vi "Check_Data.vi"(8 "error constant":errorcluster, 10 "UI Data":T2={"Script_Tree"=refnum, "Scripts"=[], "ScriptDetails"={"Script Name"="", "Steps"=[]}, "Current Step"={"StepName"="", "StepDetails"="", "Type"=enum."RELAY_CHANNEL_WRITE"}, "ScriptName"="", "StepName"="", "Children Symbols"=[], "Parrent Symbol"=[], "Configurations:"="", "Config"="", "Scriptno."=0, "PS_Write"={"Set_parameter"=0, "VOLTAGE"="", "CURRENT"="", "OUTPUT"=FALSE, "Delay"=FALSE, "Delay time"=0.0}, "DMM_CONFIG"={"CONFIG PARAMETER"=0, "AUTO RANGE"=FALSE, "RANGE"="", "Delay"=FALSE, "Delay time"=0.0}, "READ_DATAS"={"EQUIPMENT"=0, "PARAMETER"=0, "LSL"=0.0, "USL"=0.0, "RESULT"="", "UNIT"="", "Delay"=FALSE, "Delay time"=0.0}, "Set_Channel_Relay"={"Relay_CH_Array"=[]}, "DAQ_Config"={"AUTO RANGE"=FALSE, "CHANNEL LIST"="", "SELECT Card"=0, "SELECT SLOT"=0, "Function"=0}, "CAN_MSGs_Write"={"Scaling Factor"=1, "Physical value"=0.0, "CAN_Frames"={"CAN_ID"=0, "MSGTYPE"=128, "Payload"=[], "Length"=0}, "Offset value"=0.0, "Framing datas"=[], "CAN_Frame Enable"=FALSE, "Add Signal"=FALSE, "Delete Signal"=FALSE, "Signal Values"=[], "Time(ms)"=0.0, "Repetition"=FALSE, "Delay"=FALSE, "Delay time"=0.0}, "CAN_Read"={"Database"="", "Signal"="", "BYTES"=[], "ReadPayload"=[], "String_Data"="", "ReadValue"=0.0, "CANID"=0, "SERVICE ID"=0, "SUB-SERVICE ID"=0, "DELAY "=FALSE, "Delay time(ms)"=0.0}, "Camera"={"Trigger"=FALSE, "Prog No."="", "Delay"=FALSE, "Delay time"=0.0, "Storage"="", "Col no."="", "Row no."=""}, "Tab Control"=refnum, "MCU Flashing"={"Result Path"=path "", "Result"=""}, "Noeway_Flashing"={"Neoway_Firmware"=path "", "RESULT STRING"="", "Delay"=FALSE, "Delay time"=0.0}, "SSL"={"SSL_EXE"=path "", "RESULT STRING"="", "Delay"=FALSE, "Delay time"=0.0}} {"CAN_Read"."SUB-SERVICE ID" format="%.0x"; "CAN_Read"."SERVICE ID" format="%.0x"; "CAN_Read"."CANID" format="%.0x"; "CAN_Read"."ReadPayload" format="%.0x"; "CAN_MSGs_Write"."CAN_Frames"."Payload" format="%.0x"; "CAN_MSGs_Write"."CAN_Frames"."MSGTYPE" items=["STATUS"=128, "EXTENDED"=2, "RTR"=1, "DATA MSG"=0]; "CAN_MSGs_Write"."CAN_Frames"."CAN_ID" format="%.0x"; "DAQ_Config"."Function" items=["Voltage DC", "Voltage AC", "Current DC", "Current AC", "Resistance", "4-wire Resistance", "Diode", "Capacitance", "Temperature", "Continuity", "Frequency", "Period", "Voltage Ratio", "Digitize Voltage", "Digitize Current"]; "DAQ_Config"."SELECT SLOT" items=["Slot 1", "Slot 2"]; "DAQ_Config"."SELECT Card" items=["7708", "7700"]; "Set_Channel_Relay"."Relay_CH_Array"."OUTPUT_Relay_Channels" items=["CONN_SUPPLY_%d_FCT", "HB_CONN_%d_FCT", "L_IND_CONN_%d_FCT", "R_IND_CONN_%d_FCT", "SW1_%d_FCT", "SW2_%d_FCT", "CAN_H_%d_FCT", "CAN_L_%d_FCT", "CYLINDER_ON/OFF_%d_FCT", "SPARE_1_%d_FCT", "SPARE_2_%d_FCT", "Tower Red", "Tower Amber", "Tower Green", "Tower Buzzer", "SLIMRELAY_DUT_%d_FCT", "GND_DMM_%d_EOL", "CAN_H_RES_%d_EOL", "CAN_L_RES_%d_EOL", "L_IND_RES_%d_EOL", "R_IND_RES_%d_EOL", "HB_CONN_DMM_%d_EOL", "14V_RES_%d_EOL", "CAN_L_(DMM-)_%d_EOL", "CAN_H_%d_EOL", "CAN_L_%d_EOL", "14V_%d_EOL", "GND_%d_EOL", "HB_CONN_%d_EOL", "L_IND_%d_EOL", "R_IND_%d_EOL", "CYLINDER_DUT_%d_EOL", "CYL_PB_1_%d_EOL", "CYL_PB_2_%d_EOL", "DUT_PASS_%d_EOL", "DUT_FAIL_%d_EOL", "SPARE1_%d_EOL", "Tower Red_EOL", "Tower Amber_EOL", "Tower Green_EOL", "Tower Buzzer_EOL"]; "READ_DATAS"."PARAMETER" items=["SET_VOLTAGE", "SET_CURRENT", "OUTPUT VOLTAGE", "OUTPUT CURRENT", "RESISTANCE", "OUTPUT POWER", "CAMERA", "SSL_Check"]; "READ_DATAS"."EQUIPMENT" items=["POWER SUPPLY", "DMM", "DAQ", "CAMERA"]; "DMM_CONFIG"."CONFIG PARAMETER" items=["VOLTAGE", "CURRENT", "RESISTANCE", "POWER"]; "PS_Write"."Set_parameter" items=["Set_Voltage", "Set_current", "Output"]}) -> (0 "error constant 2":errorcluster, 3 "Fail?":bool)   [LabVIEW 2024, in "Setting_Screen.lvlib"]
uses:
  Setting_Screen.lvlib
  controls/Setting_Screen UI Data.ctl
  ScriptDetails.ctl
  CurrentStep.ctl
  StepType.ctl
  PS_WRITE.ctl
  PS_set.ctl
  DMM_CONFIG.ctl
  READ_DATAS.ctl
  READ_EQP.ctl
  READ_PARA.ctl
  Relay_Channel_Array.ctl
  Common_plc_DOs.ctl
  DAQ_Config.ctl
  PCANusb_DTU/support/CAN_MSGs.ctl
  PCANusb_DTU/support/CAN_Frames_ctrl.ctl
  PCANusb_DTU/support/Framing datas.ctl
  PCANusb_DTU/support/CAN_Read.ctl
  Camera.ctl
  Steptab.ctl
  MCU_Flashing/support/MCU_ctrl.ctl
  Neoway ctl.ctl
  SSL.ctl
  LOAD_WRITE.ctl
  PCANusb_DTU/PCANusb_DTU.lvlib
  MCU_Flashing/MCU_Flashing.lvlib
panel:
  out "Relay_CH_Array":cluster{"OUTPUT_PLC":T1, "On/Off":bool}[](array[cluster]) {"OUTPUT_PLC" items=["CONN_SUPPLY_%d_FCT", "HB_CONN_%d_FCT", "L_IND_CONN_%d_FCT", "R_IND_CONN_%d_FCT", "SW1_%d_FCT", "SW2_%d_FCT", "CAN_H_%d_FCT", "CAN_L_%d_FCT", "CYLINDER_ON/OFF_%d_FCT", "SPARE_1_%d_FCT", "SPARE_2_%d_FCT", "Tower Red", "Tower Amber", "Tower Green", "Tower Buzzer", "SLIMRELAY_DUT_%d_FCT", "GND_DMM_%d_EOL", "CAN_H_RES_%d_EOL", "CAN_L_RES_%d_EOL", "L_IND_RES_%d_EOL", "R_IND_RES_%d_EOL", "HB_CONN_DMM_%d_EOL", "14V_RES_%d_EOL", "CAN_L_(DMM-)_%d_EOL", "CAN_H_%d_EOL", "CAN_L_%d_EOL", "14V_%d_EOL", "GND_%d_EOL", "HB_CONN_%d_EOL", "L_IND_%d_EOL", "R_IND_%d_EOL", "CYLINDER_DUT_%d_EOL", "CYL_PB_1_%d_EOL", "CYL_PB_2_%d_EOL", "DUT_PASS_%d_EOL", "DUT_FAIL_%d_EOL", "SPARE1_%d_EOL", "Tower Red_EOL", "Tower Amber_EOL", "Tower Green_EOL", "Tower Buzzer_EOL"]}
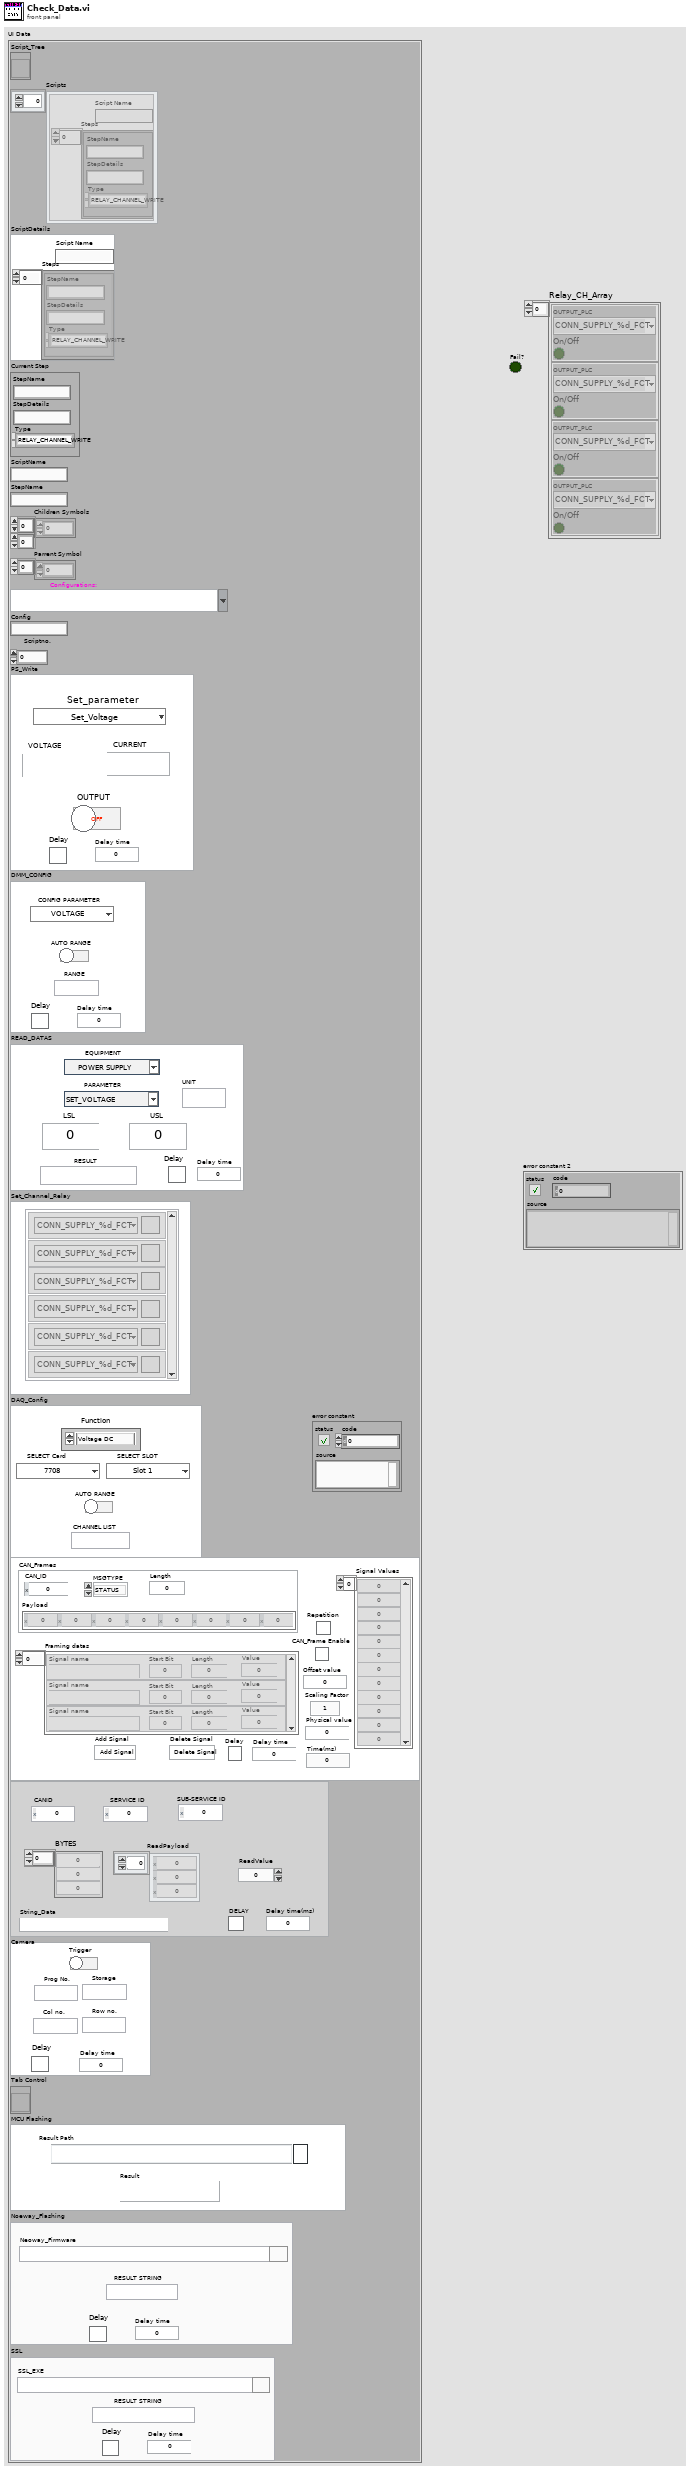
[diagram p1: front panel]
types:
  T1 = typedef "Setting_Screen.lvlib/Common_plc_DOs.ctl" = u16
  T2 = typedef "Setting_Screen.lvlib/Setting_Screen UI Data.ctl" = cluster{"Script_Tree":refnum<vi>, "Scripts":T3[], "ScriptDetails":T3, "Current Step":T4, "ScriptName":string, "StepName":string, "Children Symbols":i32[][], "Parrent Symbol":i32[], "Configurations:":string, "Config":string, "Scriptno.":i32, "PS_Write":T6, "DMM_CONFIG":T8, "READ_DATAS":T9, "Set_Channel_Relay":T12, "DAQ_Config":T13, "CAN_MSGs_Write":T14, "CAN_Read":T17, "Camera":T18, "Tab Control":refnum<vi>, "MCU Flashing":T19, "Noeway_Flashing":T20, "SSL":T21}
  T3 = typedef "Setting_Screen.lvlib/ScriptDetails.ctl" = cluster{"Script Name":string, "Steps":T4[]}
  T4 = typedef "Setting_Screen.lvlib/CurrentStep.ctl" = cluster{"StepName":string, "StepDetails":string, "Type":T5}
  T5 = typedef "Setting_Screen.lvlib/StepType.ctl" = enum16{"RELAY_CHANNEL_WRITE", "PS_WRITE", "READ_DATA", "DMM_CONFIG", "DAQ_CONFIG", "PCAN_Read", "PCAN_Write", "Camera", "MCU_Flashing", "Noeway_Flashing", "SSL_Certification"}
  T6 = typedef "Setting_Screen.lvlib/PS_WRITE.ctl" = cluster{"Set_parameter":T7, "VOLTAGE":string, "CURRENT":string, "OUTPUT":bool, "Delay":bool, "Delay time":dbl}
  T7 = typedef "Setting_Screen.lvlib/PS_set.ctl" = u16
  T8 = typedef "Setting_Screen.lvlib/DMM_CONFIG.ctl" = cluster{"CONFIG PARAMETER":u16, "AUTO RANGE":bool, "RANGE":string, "Delay":bool, "Delay time":dbl}
  T9 = typedef "Setting_Screen.lvlib/READ_DATAS.ctl" = cluster{"EQUIPMENT":T10, "PARAMETER":T11, "LSL":dbl, "USL":dbl, "RESULT":string, "UNIT":string, "Delay":bool, "Delay time":dbl}
  T10 = typedef "Setting_Screen.lvlib/READ_EQP.ctl" = u16
  T11 = typedef "Setting_Screen.lvlib/READ_PARA.ctl" = u16
  T12 = typedef "Setting_Screen.lvlib/Relay_Channel_Array.ctl" = cluster{"Relay_CH_Array":cluster{"OUTPUT_Relay_Channels":T1, "On/Off":bool}[]}
  T13 = typedef "Setting_Screen.lvlib/DAQ_Config.ctl" = cluster{"AUTO RANGE":bool, "CHANNEL LIST":string, "SELECT Card":u16, "SELECT SLOT":u16, "Function":i32}
  T14 = typedef "PCANusb_DTU.lvlib/CAN_MSGs.ctl" = cluster{"Scaling Factor":u16, "Physical value":dbl, "CAN_Frames":T15, "Offset value":dbl, "Framing datas":T16[], "CAN_Frame Enable":bool, "Add Signal":bool, "Delete Signal":bool, "Signal Values":dbl[], "Time(ms)":dbl, "Repetition":bool, "Delay":bool, "Delay time":dbl}
  T15 = typedef "PCANusb_DTU.lvlib/CAN_Frames_ctrl.ctl" = cluster{"CAN_ID":u32, "MSGTYPE":u8, "Payload":u8[], "Length":u8}
  T16 = typedef "PCANusb_DTU.lvlib/Framing datas.ctl" = cluster{"Signal name":string, "Start Bit":u8, "Length":u8, "Value":u16}
  T17 = typedef "PCANusb_DTU.lvlib/CAN_Read.ctl" = cluster{"Database":refnum<k21>, "Signal":refnum<k21>, "BYTES":u32[], "ReadPayload":u8[], "String_Data":string, "ReadValue":dbl, "CANID":u32, "SERVICE ID":u32, "SUB-SERVICE ID":u32, "DELAY ":bool, "Delay time(ms)":dbl}
  T18 = typedef "Setting_Screen.lvlib/Camera.ctl" = cluster{"Trigger":bool, "Prog No.":string, "Delay":bool, "Delay time":dbl, "Storage":string, "Col no.":string, "Row no.":string}
  T19 = typedef "MCU_Flashing.lvlib/MCU_ctrl.ctl" = cluster{"Result Path":path, "Result":string}
  T20 = typedef "Neoway ctl.ctl" = cluster{"Neoway_Firmware":path, "RESULT STRING":string, "Delay":bool, "Delay time":dbl}
  T21 = typedef "SSL.ctl" = cluster{"SSL_EXE":path, "RESULT STRING":string, "Delay":bool, "Delay time":dbl}
  T22 = cluster{"OUTPUT_Relay_Channels":T1, "On/Off":bool}[]
  T23 = typedef "Setting_Screen.lvlib/LOAD_WRITE.ctl" = cluster{"Set_parameter":T7, "VOLTAGE":string, "CURRENT":string, "OUTPUT":bool}
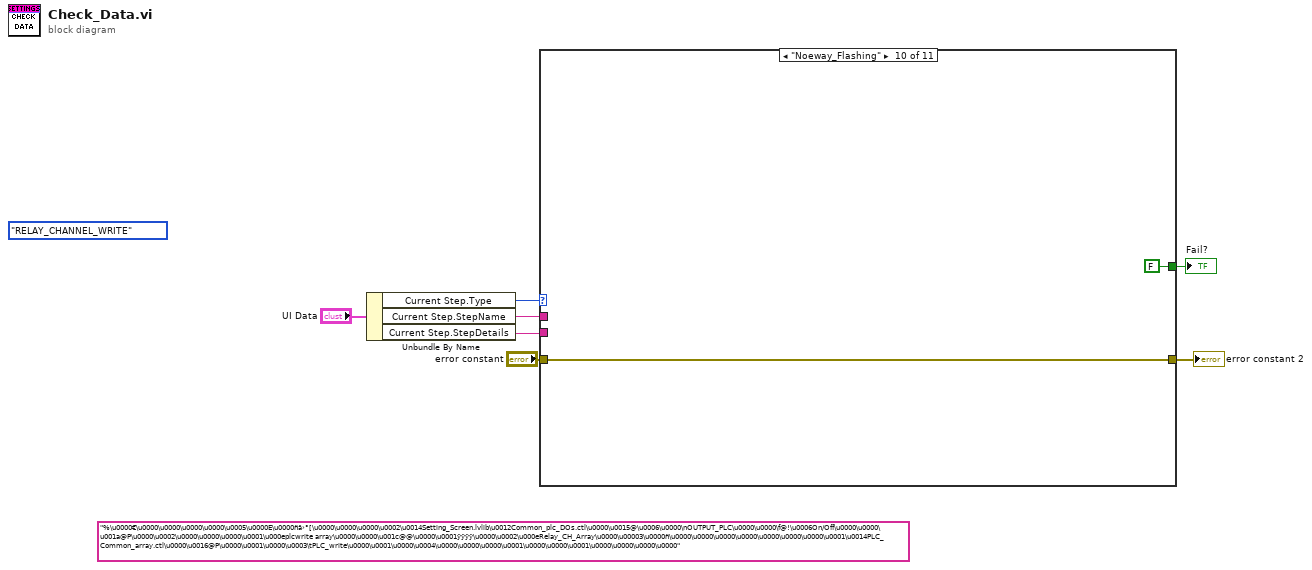
[diagram p0: block diagram]
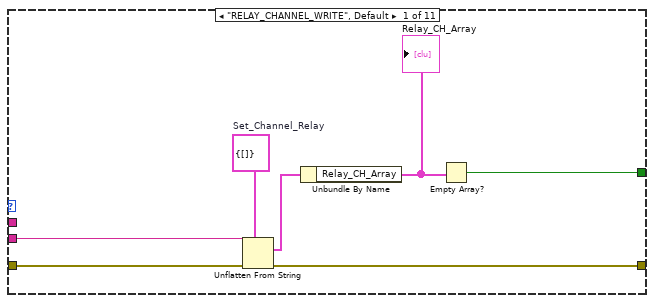
[diagram p2: hidden frame]
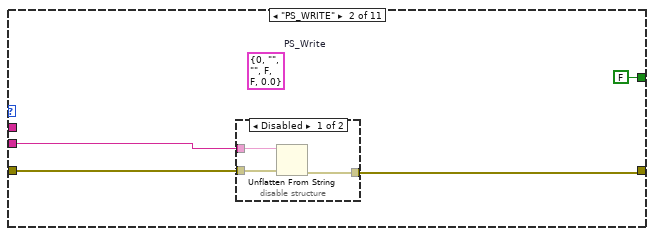
[diagram p3: hidden frame]
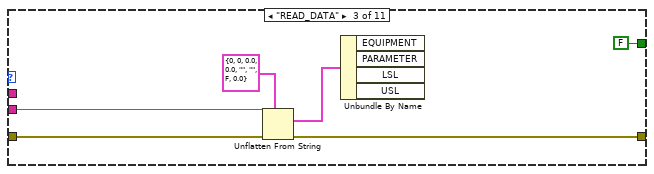
[diagram p5: hidden frame]
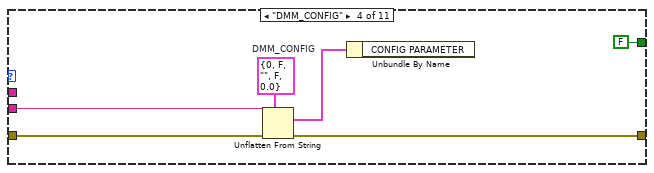
[diagram p6: hidden frame]
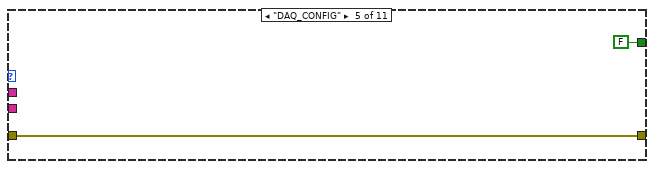
[diagram p7: hidden frame]
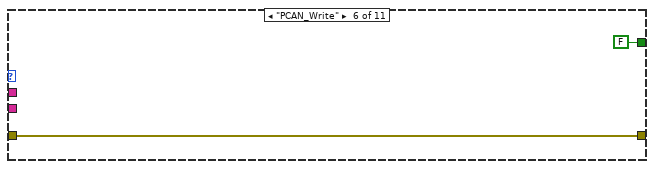
[diagram p8: hidden frame]
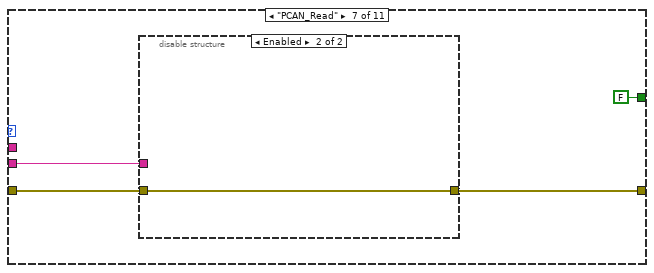
[diagram p9: hidden frame]
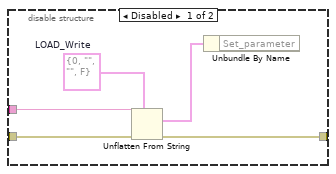
[diagram p10: hidden frame]
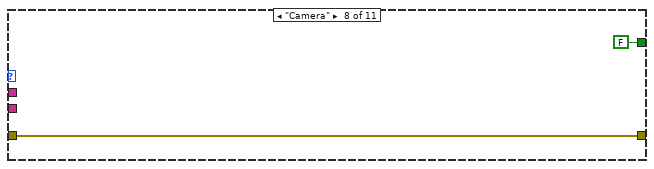
[diagram p11: hidden frame]
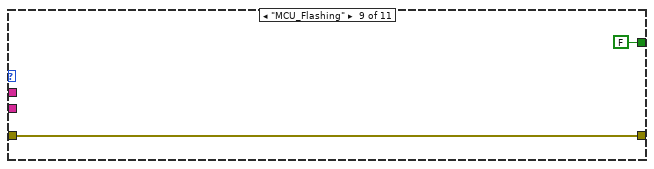
[diagram p12: hidden frame]
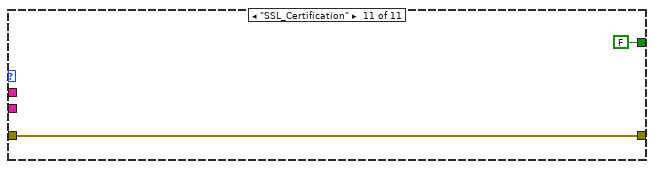
[diagram p13: hidden frame]
diagram:
  (unwired) "%\u0000€\u0000\u0000\u0000\u0000\u0005\u0000E\u0000ñä›°[\u0000\u0000\u0000\u0002\u0014Setting_Screen.lvlib\u0012Common_plc_DOs.ctl\u0000\u0015@\u0006\u0000\nOUTPUT_PLC\u0000\u0000\f@!\u0006On/Off\u0000\u0000\u001a@P\u0000\u0002\u0000\u0000\u0000\u0001\u000eplcwrite array\u0000\u0000\u001c@@\u0000\u0001ÿÿÿÿ\u0000\u0002\u000eRelay_CH_Array\u0000\u00003\u0000ñ\u0000\u0000\u0000\u0000\u0000\u0000\u0000\u0001\u0014PLC_Common_array.ctl\u0000\u0016@P\u0000\u0001\u0000\u0003\tPLC_write\u0000\u0001\u0000\u0004\u0000\u0000\u0000\u0001\u0000\u0000\u0001\u0000\u0000\u0000\u0000" ("StepDetails")
  (unwired) StepType."RELAY_CHANNEL_WRITE" ("Current Step.Type")
  n1 = Unbundle By Name("UI Data") -> ("Current Step.Type"=w2:T5, "Current Step.StepName"=w6:string, "Current Step.StepDetails"=w3:string)
  n2 = case shown="\"Noeway_Flashing\"" w2 {
    tunnel: [w13 w17 w27 w33 w36 w38 w41 w50 w52 w54 w56] -> w5
    tunnel: w6 -> [_ _ _ _ _ _ _ _ _ _ _]
    tunnel: w3 -> [w12 w16 w26 w32 _ _ w40 _ _ _ _]
    tunnel: [w9 FALSE FALSE ("empty?") FALSE ("empty?") FALSE ("empty?") FALSE ("empty?") FALSE ("empty?") FALSE ("empty?") FALSE ("empty?") FALSE ("empty?") FALSE ("empty?")] -> w4
    tunnel: "error constant" -> [w14 w18 w28 w34 w36 w38 w42 w50 w52 w54 w56]
    frame "RELAY_CHANNEL_WRITE", Default {
      w8 = T12 {"Relay_CH_Array"=[]}  # Set_Channel_Relay
      n3 = Unflatten From String(type=w8, binary string=w12, error in (no error)=w14) -> (value=w11:T12, error out=w13:errorcluster)  [unwired: 2 in, 1 out]
      n4 = Unbundle By Name(w11) -> ("Relay_CH_Array"=w10:T22)
      "Relay_CH_Array" <- w10
      n5 = Empty Array?(array=w10) -> (empty?=w9:bool)
    }
    frame "PS_WRITE" {
      (unwired) T6 {"Set_parameter"=0, "VOLTAGE"="", "CURRENT"="", "OUTPUT"=FALSE, "Delay"=FALSE, "Delay time"=0.0}  # PS_Write
      n6 = disable-structure shown="Disabled" {
        disable-tunnel: w18 -> [w21 w22]
        disable-tunnel: [w20 w22] -> w17
        disable-tunnel: w16 -> [w19 _]
        frame Disabled {
          n7 = Unflatten From String(binary string=w19, error in (no error)=w21) -> (error out=w20:errorcluster)  [unwired: 3 in, 2 out]
        }
        frame Enabled {
        }
      }
    }
    frame "READ_DATA" {
      n8 = Unflatten From String(type=T9 {"EQUIPMENT"=0, "PARAMETER"=0, "LSL"=0.0, "USL"=0.0, "RESULT"="", "UNIT"="", "Delay"=FALSE, "Delay time"=0.0} ("READ_DATAS"), binary string=w26, error in (no error)=w28) -> (value=w25:T9, error out=w27:errorcluster)  [unwired: 2 in, 1 out]
      n9 = Unbundle By Name(w25) -> ()  [unwired: 4 out]
    }
    frame "DMM_CONFIG" {
      w30 = T8 {"CONFIG PARAMETER"=0, "AUTO RANGE"=FALSE, "RANGE"="", "Delay"=FALSE, "Delay time"=0.0}  # DMM_CONFIG
      n10 = Unflatten From String(type=w30, binary string=w32, error in (no error)=w34) -> (value=w31:T8, error out=w33:errorcluster)  [unwired: 2 in, 1 out]
      n11 = Unbundle By Name(w31) -> ()  [unwired: 1 out]
    }
    frame "DAQ_CONFIG" {
    }
    frame "PCAN_Write" {
    }
    frame "PCAN_Read" {
      n12 = disable-structure shown="Enabled" {
        disable-tunnel: w42 -> [w47 w48]
        disable-tunnel: [w46 w48] -> w41
        disable-tunnel: w40 -> [w45 _]
        frame Disabled {
          w43 = T23 {"Set_parameter"=0, "VOLTAGE"="", "CURRENT"="", "OUTPUT"=FALSE}  # LOAD_Write
          n13 = Unflatten From String(type=w43, binary string=w45, error in (no error)=w47) -> (value=w44:T23, error out=w46:errorcluster)  [unwired: 2 in, 1 out]
          n14 = Unbundle By Name(w44) -> ()  [unwired: 1 out]
        }
        frame Enabled {
        }
      }
    }
    frame "Camera" {
    }
    frame "MCU_Flashing" {
    }
    frame "Noeway_Flashing" {
    }
    frame "SSL_Certification" {
    }
  }
  "error constant 2" <- w5
  "Fail?" <- w4
